vi "Load stack of I16 images with metadata from Tiff Stack file.vi"(7 "path to TIFF file":path=path "C:/Users/dmilkie/Desktop/stack.tif", 8 "error in":errorcluster, 11 "Images":T1[](array[typedef])) -> (0 "error out":errorcluster, 3 "Images dup":T1[](array[typedef]), 4 "ImageDescriptions":string[](array[string]))   [LabVIEW 2015, in "Tiff reader.lvlib"]
doc: "This .vi is taken from an online tiff reader. It is able to read 32-bit floating point .tiff images."
uses:
  Tiff reader.lvlib
  <vilib>/vision/Image Controls.llb/IMAQ Image.ctl
panel:
  out "Image #":i32
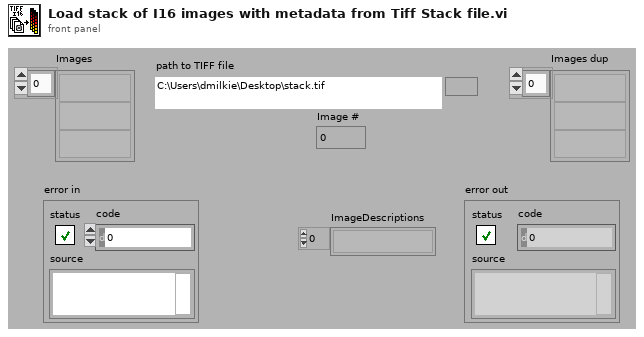
[diagram p1: front panel]
types:
  T1 = typedef "IMAQ Image.ctl" = refnum<image>
  T2 = enum16{"open", "replace", "create", "open or create", "replace or create", "replace or create with confirmation"}
  T3 = typedef "Tiff reader.lvlib/IFD Entry.ctl" = cluster{"Tag":u16, "Type":T4, "Count":u32, "Val/Offs":u32, "Is Pointer?":bool, "Byte stream index":i32}
  T4 = typedef "Tiff reader.lvlib/FieldTypes.ctl" = enum16{"NULL", "U8", "ASCII7", "U16", "U32", "RATIONAL", "SByte(I8)", "Undef(8Bit)", "I16", "I32", "SRat(4B:4B)", "SGL(4Byte)", "DBL(8Byte)"}
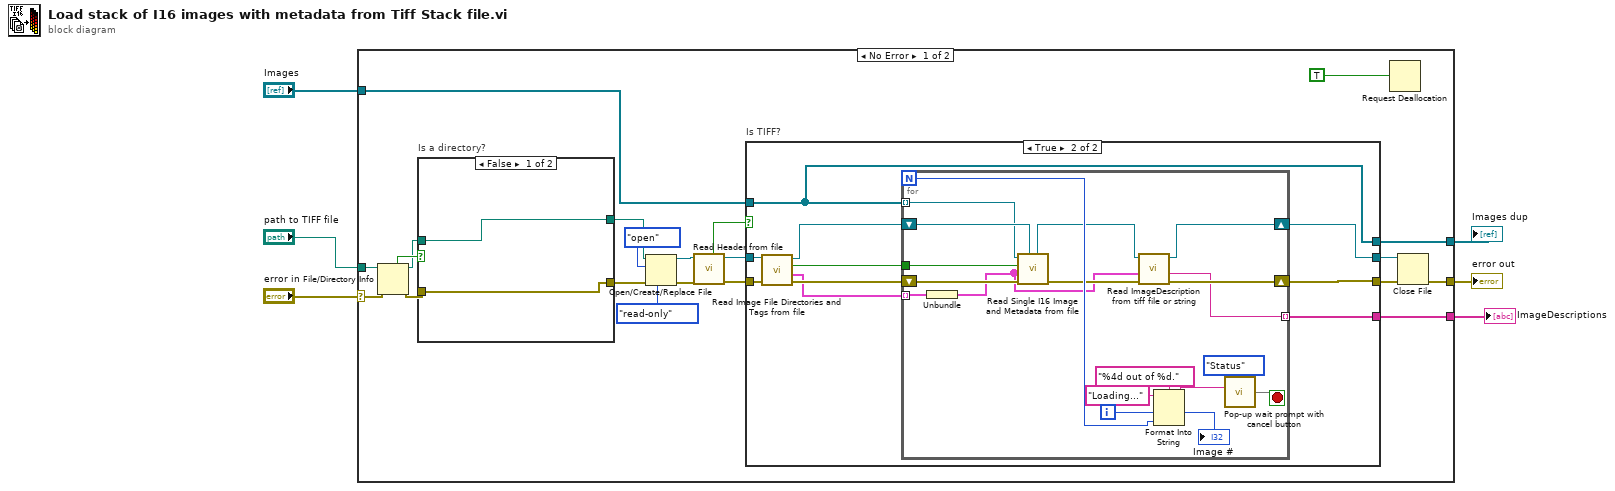
[diagram p0: block diagram]
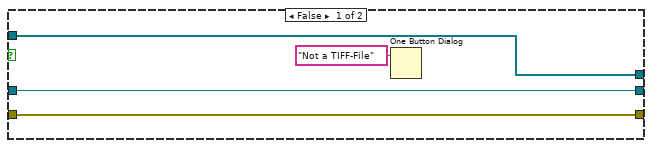
[diagram p2: hidden frame]
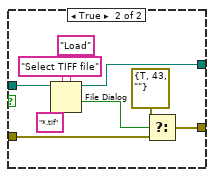
[diagram p3: hidden frame]
diagram:
  n1 = case shown="No Error" "error in" {
    selector: "error in" -> [w16 w72]
    tunnel: "path to TIFF file" -> [w26 _]
    tunnel: [w17 w71] -> w5
    tunnel: [w9 w72] -> w4
    tunnel: "Images" -> [w15 w71]
    tunnel: [w7 _] -> w1
    frame No Error {
      n2 = File/Directory Info(path=w26, error in=w16) -> (path out=w14:path, directory=w27:bool, error out=w25:errorcluster)  [unwired: 4 out]
      n3 = case "Is a directory?" shown="False" w27 {
        tunnel: w25 -> [w61 w67]
        tunnel: w14 -> [w60 w66]
        tunnel: [w61 w62] -> w20
        tunnel: [w60 w63] -> w19
        frame False {
        }
        frame True {
          n4 = File Dialog(5:"Load" ("button label"), 6:"*.tif" ("pattern"), 7:"Select TIFF file" ("prompt"), 11:w66) -> (1:w68:bool, 3:w63:path)  [unwired: 1 in, 4 out]
          n5 = Select(t=errorcluster {"status"=TRUE, "code"=43, "source"=""} ("error in (no error)"), s=w68, f=w67) -> (s? t:f=w62:errorcluster)
        }
      }
      n6 = Open/Create/Replace File(file path (use dialog)=w19, error in=w20, operation (0:open)=T2."open", access (0:read/write)=enum16{"read/write", "read-only", "write-only"}."read-only") -> (refnum out=w18:refnum<file>, error out=w21:errorcluster)  [unwired: 3 out]
      n7 = call "Read Header from file.vi"("error in"=w21, "File"=w18) -> ("error out"=w12:errorcluster, "File"=w13:refnum<file>, "isTIFF"=w11:bool)  [unwired: 5 out]
      n8 = case "Is TIFF?" shown="True" w11 {
        tunnel: [w30 w34] -> w17
        tunnel: [w29 w33] -> w10
        tunnel: w15 -> [w30 w34]
        tunnel: w13 -> [w28 w41]
        tunnel: w12 -> [w29 w40]
        tunnel: [w28 w36] -> w8
        tunnel: [_ w32] -> w7
        frame False {
          n9 = One Button Dialog(message="Not a TIFF-File") -> ()  [unwired: 2 out]
        }
        frame True {
          n10 = call "Read Image File Directories and Tags from file.vi"("error in"=w40, "File"=w41) -> ("error out"=w38:errorcluster, "Tags for each IFD"=w35:cluster{"Tags":T3[]}[], "Litt/BigEnd"=w37:bool, "File"=w39:refnum<file>)  [unwired: 2 out]
          n11 = for {
            N -> [w48]
            tunnel: w34 -> [w49] mode=indexing
            shift-right: [w44] -> w36
            shift-left: w39 -> [w50]
            tunnel: w35 -> [w59] mode=indexing
            tunnel: w37 -> [w51]
            shift-right: [w46] -> w33
            shift-left: w38 -> [w52]
            tunnel: [w42] -> w32 mode=indexing
            i -> [w54]
            stop <- w58 stop-if-true
            n12 = Unbundle(w59) -> ("Tags"=w43:T3[])
            n13 = call "Read Single I16 Image and Metadata from file.vi"("File"=w50, "error out"=w52, "Tags"=w43, "Litt/BigEnd"=w51, "Image"=w49) -> ("error out"=w47:errorcluster, "File dup"=w45:refnum<file>)  [unwired: 2 in, 3 out]
            n14 = call "Read ImageDescription from tiff file or string.vi"("error in"=w47, "DirEntries"=w43, "Tiff image stack"=w45) -> ("error out"=w46:errorcluster, "ImageDescription string"=w42:string, "Tiff image stack dup"=w44:refnum<file>)  [unwired: 5 in, 1 out]
            n15 = Format Into String(format string="%4d out of %d.", initial string="Loading...", w54, w48) -> (resulting string=w56:string)  [unwired: 1 in, 1 out]
            n16 = call "Pop-up wait prompt with cancel button.vi"(9:w56, 11:enum16{"Open", "Close", "Status", "No Change"}."Status" ("Control")) -> (1:w58)  [unwired: 1 in, 8 out]
            "Image #" <- w54
          }
        }
      }
      n17 = Request Deallocation(TRUE ("flag")) -> ()
      n18 = Close File(refnum=w8, error in=w10) -> (error out=w9:errorcluster)  [unwired: 1 out]
    }
    frame Error {
    }
  }
  "error out" <- w4
  "Images dup" <- w5
  "ImageDescriptions" <- w1
